vi "getNonOverlapIdx.vi"(8 "error in (no error)":errorcluster, 9 "Overlap Idx Array":i32[](array[numeric]), 10 "Input Idx Array":i32[](array[numeric]), 11 "MatOper in":refnum<class "MatOper.lvclass">) -> (0 "error out":errorcluster, 2 "Non-Overlap Idx Array":i32[](array[numeric]), 3 "MatOper out":refnum<class "MatOper.lvclass">)   [LabVIEW 2016, in "OfcFunc.lvlib" / "MatOper.lvclass"]
doc: "Get the non overlap index array from the input index array."
uses:
  MatOper.lvclass
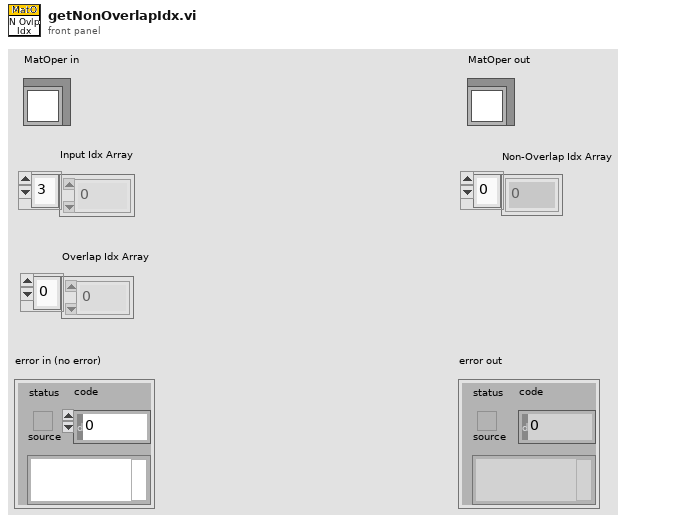
[diagram p1: front panel]
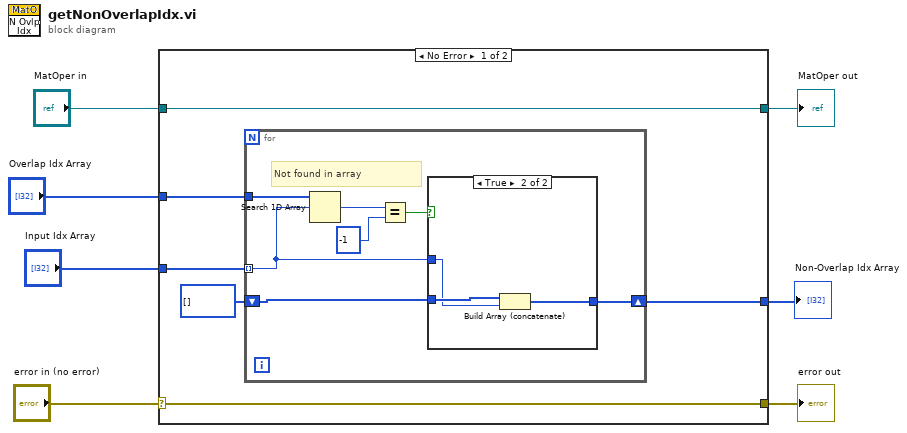
[diagram p0: block diagram]
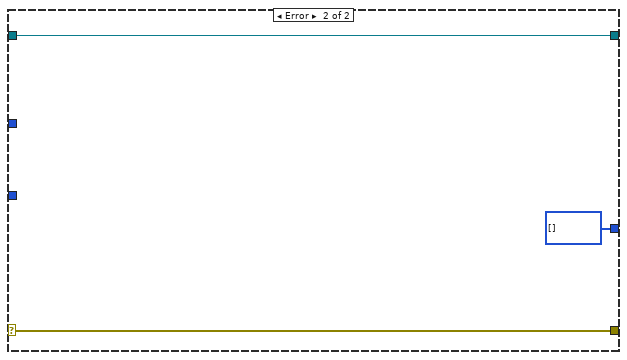
[diagram p3: hidden frame]
diagram:
  n1 = case shown="No Error" "error in (no error)" {
    selector: "error in (no error)" -> [w12 w27]
    tunnel: [w12 w27] -> w6
    tunnel: [w13 w26] -> w4
    tunnel: "MatOper in" -> [w13 w26]
    tunnel: "Input Idx Array" -> [w10 _]
    tunnel: "Overlap Idx Array" -> [w9 _]
    tunnel: [w8 i32[] []] -> w1
    frame No Error {
      n2 = for {
        tunnel: w9 -> [w20]
        tunnel: w10 -> [w16] mode=indexing
        shift-right: [w14] -> w8
        shift-left: i32[] [] -> [w15]
        # "Not found in array"
        n3 = Search 1D Array(1D array=w20, element=w16) -> (index of element=w19:i32)  [unwired: 1 in]
        n4 = Equal?(x=w19, y=-1) -> (x = y?=w17:bool)
        n5 = case shown="True" w17 {
          tunnel: w16 -> [_ w22]
          tunnel: w15 -> [w21 w24]
          tunnel: [w21 w23] -> w14
          frame False {
          }
          frame True {
            n6 = Build Array (concatenate)(w24, w22) -> (w23:i32[])
          }
        }
      }
    }
    frame Error {
    }
  }
  "error out" <- w6
  "MatOper out" <- w4
  "Non-Overlap Idx Array" <- w1
